vi "ConfigSyncInfo.vi"(8 "error in (no error)":errorcluster, 10 "SyncInfo":variant, 11 "DigitizerBase in":refnum<class "DigitizerBase.lvclass">) -> (0 "error out":errorcluster, 3 "DigitizerBase out":refnum<class "DigitizerBase.lvclass">)   [LabVIEW 2018, in "DigitizerPlugins.lvlib" / "DigitizerBase.lvclass"]
uses:
  DigitizerBase.lvclass
  DigitizerBase.lvclass/DigitizerBase.ctl
  Accessors/Write SyncInfo.vi
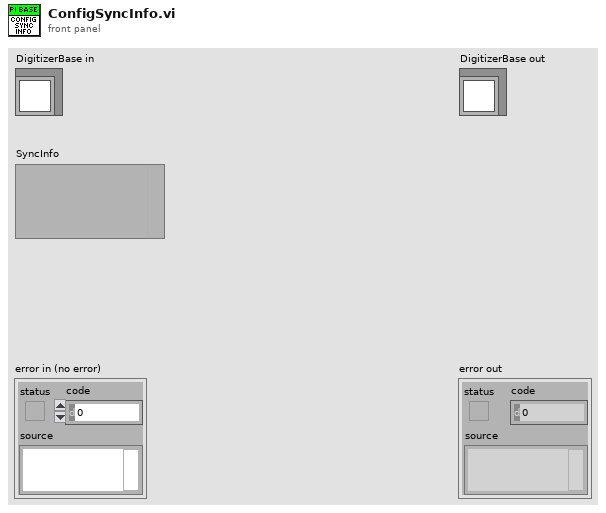
[diagram p1: front panel]
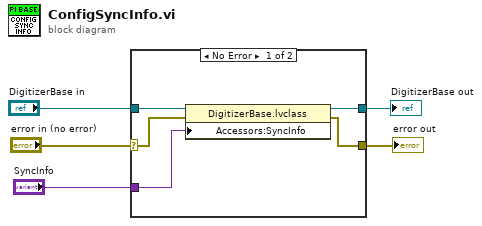
[diagram p0: block diagram]
diagram:
  n1 = case shown="No Error" "error in (no error)" {
    selector: "error in (no error)" -> [w8 w12]
    tunnel: [w7 w12] -> w4
    tunnel: [w9 w11] -> w2
    tunnel: "DigitizerBase in" -> [w10 w11]
    tunnel: "SyncInfo" -> [w6 _]
    frame No Error {
      n2 = property class="DigitizerBase.lvclass"(reference=w10, error in=w8, "Accessors:SyncInfo"=w6) -> (reference out=w9:refnum<class "DigitizerBase.lvclass">, error out=w7:errorcluster)
    }
    frame Error {
    }
  }
  "error out" <- w4
  "DigitizerBase out" <- w2
